vi "DSF.Engine.Builder.Buffer.Build.vi"(6 "VS Channel Buffer in":dbl[](array[numeric]), 8 "error in (no error)":errorcluster, 10 "command":T3, 11 "Builder in":refnum<class "DSF.Engine.Builder.lvclass">) -> (0 "error out":errorcluster, 2 "response":T1, 3 "Builder out":refnum<class "DSF.Engine.Builder.lvclass">, 4 "VS Channel Buffer out":dbl[](array[numeric]))   [LabVIEW 2016, in "DSF.Engine.lvlib" / "DSF.Engine.Builder.lvclass"]
uses:
  DSF.Engine.Builder.lvclass
  Interface/DSF.Engine.Interface.Builder.Command Data.ctl
  Interface/DSF.Engine.Interface.Builder.Command.ctl
  Interface/DSF.Engine.Interface.Builder.Response Data.ctl
  Interface/DSF.Engine.Interface.Builder.Response.ctl
  Interface/DSF.Engine.Interface.Builder.lvclass
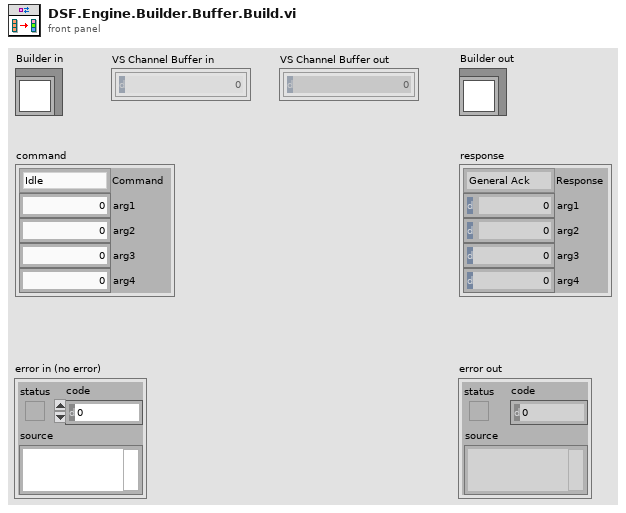
[diagram p1: front panel]
types:
  T1 = typedef "DSF.Engine.lvlib/DSF.Engine.Interface.Builder.lvclass/DSF.Engine.Interface.Builder.Response Data.ctl" = cluster{"Response":T2, "arg1":i32, "arg2":i32, "arg3":i32, "arg4":i32}
  T2 = typedef "DSF.Engine.lvlib/DSF.Engine.Interface.Builder.lvclass/DSF.Engine.Interface.Builder.Response.ctl" = enum8{"General Ack", "Initialize Complete", "Build Complete", "Parse Complete", "Shutdown Ack"}
  T3 = typedef "DSF.Engine.lvlib/DSF.Engine.Interface.Builder.lvclass/DSF.Engine.Interface.Builder.Command Data.ctl" = cluster{"Command":T4, "arg1":i32, "arg2":i32, "arg3":i32, "arg4":i32}
  T4 = typedef "DSF.Engine.lvlib/DSF.Engine.Interface.Builder.lvclass/DSF.Engine.Interface.Builder.Command.ctl" = enum8{"Idle", "Initialize", "Build Buffer", "Parse Buffer", "Shutdown"}
  T5 = typedef "DSF.Engine.lvlib/DSF.Engine.Builder.lvclass/DSF.Engine.Builder.Command.Build-Parse.ctl" = cluster{"unused":u8, "Plugin ID":i32, "Transfer Group ID":i32, "Transfer ID":i32, "unused":i32}
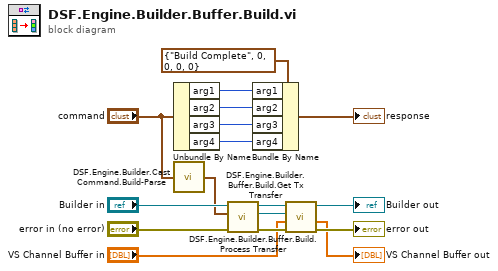
[diagram p0: block diagram]
diagram:
  n1 = Unbundle By Name("command") -> ("arg1"=w15:i32, "arg2"=w16:i32, "arg3"=w13:i32, "arg4"=w12:i32)
  n2 = call "DSF.Engine.Builder.Cast Command.Build-Parse.vi"("command"="command") -> ("build/parse command"=w10:T5)
  n3 = call "DSF.Engine.Builder.Buffer.Build.Get Tx Transfer.vi"("error in (no error)"="error in (no error)", "build/parse command"=w10, "Builder in"="Builder in") -> ("error out"=w3:errorcluster, "Transfer"=w5:refnum<class "DSF.Engine.Transfer.lvclass">, "Builder out"=w9:refnum<class "DSF.Engine.Builder.lvclass">)  [unwired: 6 in]
  n4 = Bundle By Name(cluster=T1 {"Response"=enum."Build Complete", "arg1"=0, "arg2"=0, "arg3"=0, "arg4"=0} ("response"), "arg1"=w15, "arg2"=w16, "arg3"=w13, "arg4"=w12) -> (→"response":T1)
  n5 = call "DSF.Engine.Builder.Buffer.Build.Process Transfer.vi"("error in (no error)"=w3, "VS Channel Buffer in"="VS Channel Buffer in", "Transfer"=w5, "Builder in"=w9) -> ("error out"=→"error out":errorcluster, "VS Channel Buffer out"=→"VS Channel Buffer out":dbl[], "Builder out"=→"Builder out":refnum<class "DSF.Engine.Builder.lvclass">)  [unwired: 5 in]
